vi "Teleop.vi"(10 "Match Info":T1={"Autonomous Elapsed Seconds"=0.0, "TeleOp Elapsed Seconds"=0.0, "Disabled Elapsed Seconds"=0.0, "Visited Autonomous"=FALSE, "Visited TeleOp"=FALSE, "Visited Disabled"=FALSE, "Autonomous Settings"={"Autonomous Style"=enum."Independent", "VI Refnum"=refnum}}, 11 "Call Context":T2) -> ()   [LabVIEW 2016]
doc: "This VI is called for each TeleOp packet received from the DS where the robot is not disabled. It is often used to read from the joysticks and update I/O or to update setpoints for timed control loops. It should complete and return within 20 milliseconds or it may miss DS packets."
uses:
  <vilib>/Rock Robotics/WPI/DriverStation/WPI_DriverStationDerivedRobotMode.ctl
  <vilib>/Rock Robotics/WPI/DriverStation/WPI_DriverStationMatch Info.ctl
  <vilib>/Rock Robotics/WPI/Solenoid/WPI_SolenoidValue.ctl
  <vilib>/Rock Robotics/WPI/Utilities/WPI_GetSetVariantRefNum.vi
  <vilib>/Rock Robotics/WPI/Solenoid/WPI_SolenoidSetEnum.vi
panel:
  out "Gyro Angle":dbl format="%#_13g"
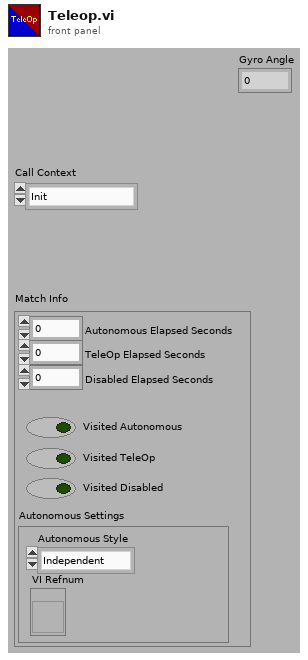
[diagram p1: front panel]
types:
  T1 = typedef "WPI_DriverStationMatch Info.ctl" = cluster{"Autonomous Elapsed Seconds":dbl, "TeleOp Elapsed Seconds":dbl, "Disabled Elapsed Seconds":dbl, "Visited Autonomous":bool, "Visited TeleOp":bool, "Visited Disabled":bool, "Autonomous Settings":cluster{"Autonomous Style":enum16{"Iterative", "Independent"}, "VI Refnum":refnum<vi>}}
  T2 = typedef "WPI_DriverStationDerivedRobotMode.ctl" = enum16{"Init", "Execute", "Stop"}
  T3 = typedef "WPI_SolenoidValue.ctl" = enum16{"Off", "On", "Forward", "Reverse"}
  T4 = typedef "WPI_AccelerometerDevRef.ctl" = cluster{"DevStatus":errorcluster, "Scaling":T5, "Analog Channels":T6, "I2C Bus":T8, "SPI Bus":T9, "Accel Range":T10, "ADXL Axes":T11, "Handle":i32, "Device Address":u8, "Accel Type":enum16{"Analog", "ADXL345 I2C", "ADXL345 SPI", "Internal", "ADXL362 SPI"}}
  T5 = typedef "WPI_AccelerometerScaling.ctl" = cluster{"Gain (VoltsPerG)":dbl, "Center Voltage":dbl}
  T6 = typedef "WPI_AccelerometerAnalogChannels.ctl" = cluster{"X-Axis":T7, "Y-Axis":T7, "Z-Axis":T7}
  T7 = typedef "FPGA_AIChannel.ctl" = enum8{"AI 0", "AI 1", "AI 2", "AI 3", "AI MXP 0", "AI MXP 1", "AI MXP 2", "AI MXP 3", "Invalid"}
  T8 = typedef "i2c_bus.ctl" = enum16{"I2C On-Board", "I2C MXP", "Invalid"}
  T9 = typedef "spi_bus.ctl" = enum16{"SPI On-Board, CS0", "SPI On-Board, CS1", "SPI On-Board, CS2", "SPI On-Board, CS3", "SPI MXP", "Invalid"}
  T10 = typedef "ADXL345 Range.ctl" = u8
  T11 = typedef "WPI_AccelerometerADXL345 Axes.ctl" = cluster{"X-Axis":bool, "Y-Axis":bool, "Z-Axis":bool}
  T12 = cluster{"X-Axis":dbl, "Y-Axis":dbl, "Z-Axis":dbl}
  T13 = typedef "WPI_JoystickDevRef.ctl" = cluster{"Device":T14}
  T14 = typedef "WPI_JoystickDeviceEnum.ctl" = enum16{"USB 0", "USB 1", "USB 2", "USB 3", "USB 4", "USB 5"}
  T15 = typedef "WPI_GyroDevRef.ctl" = cluster{"DevStatus":errorcluster, "Analog Channel":T7, "Offset":dbl, "Gain (VoltsPerDegree/Second)":dbl, "Gyro Type":enum16{"Analog", "XRS450"}, "Handle":i32, "SPI Bus":T9, "Device Found":bool, "Sample Rate":dbl, "Calibrate On Open":bool}
  T16 = typedef "WPI_MotorControlDeviceRef.ctl" = cluster{"DeviceStatus":errorcluster, "Type":T17, "PWM":cluster{"PWM Channel":T18, "DeadBand":T19}, "CAN":cluster{"Device Number":u8, "SetOutput VI Ref":variant, "GetOutput VI Ref":variant, "Enable VI Ref":variant, "Disable VI Ref":variant, "Data":variant}, "Invert":bool}
  T17 = typedef "WPI_MotorControlType.ctl" = enum16{"PWM", "CAN"}
  T18 = typedef "FPGA_DIOPWMChannel.ctl" = enum8{"PWM 0", "PWM 1", "PWM 2", "PWM 3", "PWM 4", "PWM 5", "PWM 6", "PWM 7", "PWM 8", "PWM 9", "PWM MXP 0", "PWM MXP 1", "PWM MXP 2", "PWM MXP 3", "PWM MXP 4", "PWM MXP 5", "PWM MXP 6", "PWM MXP 7", "PWM MXP 8", "PWM MXP 9", "Invalid"}
  T19 = typedef "WPI_PWMDeadband.ctl" = cluster{"Name":string, "maxPositivePwm":i32, "minPositivePwm":i32, "centerPwm":i32, "maxNegativePwm":i32, "minNegativePwm":i32, "angularRange":u16}
  T20 = typedef "WPI_SolenoidDevRef.ctl" = cluster{"DevStatus":errorcluster, "Pneumatics Control Module":u8, "Forward Solenoid Channel":T21, "Reverse Solenoid Channel":T21}
  T21 = typedef "WPI_SolenoidChannel.ctl" = enum8{"Solenoid 0", "Solenoid 1", "Solenoid 2", "Solenoid 3", "Solenoid 4", "Solenoid 5", "Solenoid 6", "Solenoid 7", "Invalid"}
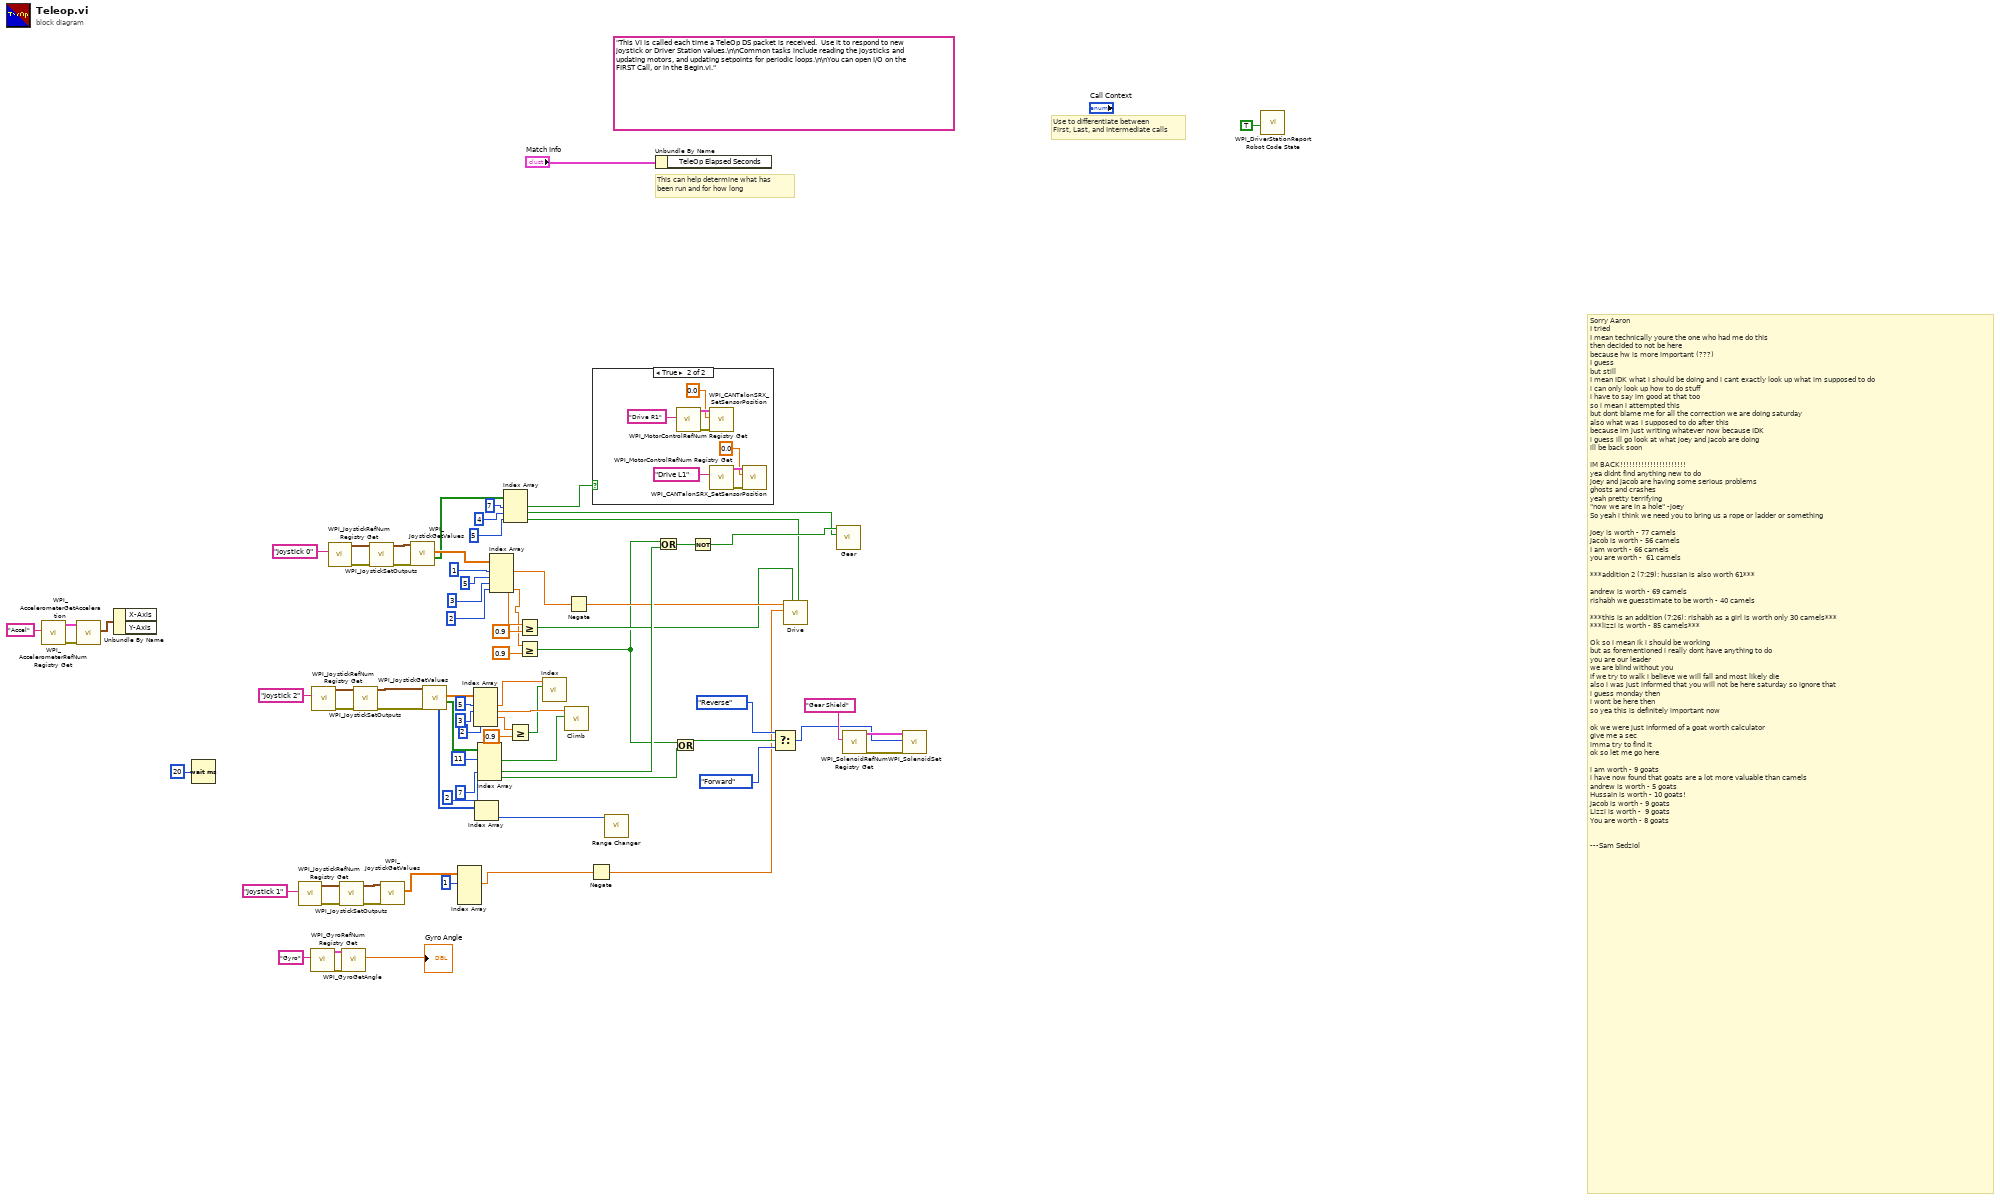
[diagram p0: block diagram]
diagram:
  (unwired) "This VI is called each time a TeleOp DS packet is received.  Use it to respond to new joystick or Driver Station values.\n\nCommon tasks include reading the joysticks and updating motors, and updating setpoints for periodic loops.\n\nYou can open I/O on the FIRST Call, or in the Begin.vi."
  # "Sorry Aaron\nI tried\nI mean technically youre the one who had me do this\nthen decided to not be here\nbecause hw is more important (???)\nI guess\nbut still\nI mean IDK what i should be doing and i cant exactly look up what im supposed to do\ni can only look up how to do stuff\ni have to say im good at that too\nso i mean i attempted this\nbut dont blame me for all the correction we are doing saturday\nalso what was i supposed to do after this\nbecause im just writing whatever now because IDK\ni guess ill go look at what joey and jacob are doing\nill be back soon\n\nIM BACK!!!!!!!!!!!!!!!!!!!!!!\nyea didnt find anything new to do\njoey and jacob are having some serious problems\nghosts and crashes\nyeah pretty terrifying\n\"now we are in a hole\" -joey\nSo yeah i think we need you to bring us a rope or ladder or something\n\nJoey is worth - 77 camels\nJacob is worth - 56 camels\nI am worth - 66 camels\nyou are worth -  61 camels \n\n***addition 2 (7:29): hussian is also worth 61***\n\nandrew is worth - 69 camels\nrishabh we guesstimate to be worth - 40 camels\n\n***this is an addition (7:26): rishabh as a girl is worth only 30 camels***\n***lizzi is worth - 85 camels***\n\nOk so i mean ik i should be working\nbut as forementioned i really dont have anything to do\nyou are our leader\nwe are blind without you\nif we try to walk i believe we will fall and most likely die\nalso i was just informed that you will not be here saturday so ignore that\ni guess monday then\ni wont be here then\nso yea this is definitely important now\n\nok we were just informed of a goat worth calculator\ngive me a sec \nimma try to find it\nok so let me go here\n\ni am worth - 9 goats\ni have now found that goats are a lot more valuable than camels\nandrew is worth - 5 goats\nHussain is worth - 10 goats! \nJacob is worth - 9 goats\nLizzi is worth -  9 goats\nYou are worth - 8 goats\n\n\n---Sam Sedziol"
  # "Use to differentiate between\nFirst, Last, and Intermediate calls"
  # "This can help determine what has\nbeen run and for how long"
  n1 = call <vilib>:"WPI_AccelerometerRefNum Registry Get.vi"("refnum name"="Accel") -> ("error out"=w21:errorcluster, "AccelerometerDevRef"=w20:T4)  [unwired: 9 in]
  n2 = call <vilib>:"WPI_AccelerometerGetAcceleration.vi"("error in"=w21, "AccelerometerDevRef"=w20) -> ("Accelerations"=w22:T12)  [unwired: 7 in, 2 out]
  n3 = Unbundle By Name(w22) -> ()  [unwired: 2 out]
  n4 = Wait (ms)(milliseconds to wait=u32 20) -> ()  [unwired: 1 out]
  n5 = call <vilib>:"WPI_JoystickRefNum Registry Get.vi"("refnum name"="Joystick 1") -> ("error out"=w7:errorcluster, "JoystickDevRef"=w9:T13)  [unwired: 1 in, 8 out]
  n6 = call <vilib>:"WPI_GyroRefNum Registry Get.vi"("refnum name"="Gyro") -> ("error out"=w61:errorcluster, "GyroDevRef"=w60:T15)  [unwired: 9 in]
  n7 = call <vilib>:"WPI_JoystickRefNum Registry Get.vi"("refnum name"="Joystick 2") -> ("error out"=w15:errorcluster, "JoystickDevRef"=w18:T13)  [unwired: 1 in, 8 out]
  n8 = call <vilib>:"WPI_JoystickRefNum Registry Get.vi"("refnum name"="Joystick 0") -> ("error out"=w12:errorcluster, "JoystickDevRef"=w14:T13)  [unwired: 1 in, 8 out]
  n9 = call <vilib>:"WPI_JoystickSetOutputs.vi"("error in (no error)"=w7, "JoystickDevRef"=w9) -> ("error out"=w6:errorcluster, "JoystickDevRef"=w8:T13)  [unwired: 8 in]
  n10 = call <vilib>:"WPI_GyroGetAngle.vi"("error in (no error)"=w61, "GyroDevRef"=w60) -> ("Angle"=→"Gyro Angle":dbl)  [unwired: 6 in, 3 out]
  n11 = call <vilib>:"WPI_JoystickSetOutputs.vi"("error in (no error)"=w15, "JoystickDevRef"=w18) -> ("error out"=w16:errorcluster, "JoystickDevRef"=w17:T13)  [unwired: 8 in]
  n12 = call <vilib>:"WPI_JoystickSetOutputs.vi"("error in (no error)"=w12, "JoystickDevRef"=w14) -> ("error out"=w11:errorcluster, "JoystickDevRef"=w13:T13)  [unwired: 8 in]
  n13 = call <vilib>:"WPI_JoystickGetValues.vi"("error in (no error)"=w6, "JoystickDevRef"=w8) -> ("Axes"=w5:dbl[])  [unwired: 5 in, 4 out]
  n14 = call <vilib>:"WPI_JoystickGetValues.vi"("error in (no error)"=w11, "JoystickDevRef"=w13) -> ("Buttons"=w70:bool[], "Axes"=w74:dbl[])  [unwired: 5 in, 3 out]
  n15 = call <vilib>:"WPI_JoystickGetValues.vi"("error in (no error)"=w16, "JoystickDevRef"=w17) -> ("Buttons"=w71:bool[], "Axes"=w72:dbl[], "POVs"=w50:i16[])  [unwired: 5 in, 2 out]
  n16 = Index Array(array=w5, index #1=1 ("index")) -> (element #1=w3:dbl)  [unwired: 3 in, 3 out]
  n17 = Index Array(array=w72, index #1=5 ("index"), index #2=3 ("index"), index #3=2 ("index")) -> (element #1=w57:dbl, element #2=w66:dbl, element #3=w25:dbl)  [unwired: 1 in, 1 out]
  n18 = Index Array(array=w50) -> (element=w49:i16)  [unwired: 1 in]
  n19 = Index Array(array=w71, index #1=11 ("index"), index #3=7 ("index"), index #4=2) -> (element #1=w54:bool, element #3=w55:bool, element #4=w37:bool)  [unwired: 1 in, 1 out]
  n20 = Index Array(array=w74, index #1=1 ("index"), index #2=5 ("index"), index #3=3 ("index"), index #4=2 ("index")) -> (element #1=w41:dbl, element #3=w35:dbl, element #4=w30:dbl)  [unwired: 1 out]
  n21 = Index Array(array=w70, index #1=7 ("index"), index #2=4 ("index"), index #3=5 ("index")) -> (element #1=w68:bool, element #2=w1:bool, element #3=w27:bool)
  n22 = Greater Or Equal?(x=w25, y=0.9) -> (x >= y?=w23:bool)
  n23 = Greater Or Equal?(x=w35, y=0.9) -> (x >= y?=w31:bool)
  n24 = Greater Or Equal?(x=w30, y=0.9) -> (x >= y?=w29:bool)
  n25 = call "Index.vi"("Shoot"=w23, "Output 2"=w57) -> ()  [unwired: 10 in]
  n26 = call "Climb.vi"("Backwards?"=w54, "Effort"=w66) -> ()  [unwired: 10 in]
  n27 = Negate(x=w41) -> (-x=w36:dbl)
  n28 = Negate(x=w3) -> (-x=w2:dbl)
  n29 = case shown="True" w68 {
    frame False {
    }
    frame True {
      n30 = call <vilib>:"WPI_MotorControlRefNum Registry Get.vi"("refnum name"="Drive R1") -> ("error out"=w80:errorcluster, "MotorControlDevRef"=w79:T16)  [unwired: 9 in]
      n31 = call <vilib>:"WPI_CANTalonSRX_SetSensorPosition.vi"("error in (no error)"=w80, "New Sensor Position"=0.0, "CAN Talon SRX Ref"=w79) -> ()  [unwired: 7 in, 2 out]
      n32 = call <vilib>:"WPI_MotorControlRefNum Registry Get.vi"("refnum name"="Drive L1") -> ("error out"=w82:errorcluster, "MotorControlDevRef"=w83:T16)  [unwired: 9 in]
      n33 = call <vilib>:"WPI_CANTalonSRX_SetSensorPosition.vi"("error in (no error)"=w82, "New Sensor Position"=0.0, "CAN Talon SRX Ref"=w83) -> ()  [unwired: 7 in, 2 out]
    }
  }
  n34 = call "Range Changer.vi"("POV"=w49) -> ()  [unwired: 10 in, 1 out]
  n35 = Unbundle By Name("Match Info") -> ()  [unwired: 1 out]
  n36 = Or(x=w29, y=w55) -> (x .or. y?=w62:bool)
  n37 = Or(x=w29, y=w37) -> (x .or. y?=w38:bool)
  n38 = Not(x=w62) -> (.not. x?=w52:bool)
  n39 = Select(t=WPI_SolenoidValue."Reverse" ("Value"), s=w38, f=WPI_SolenoidValue."Forward" ("Value")) -> (s? t:f=w42:T3)
  n40 = call "Drive.vi"("SwitchDir"=w27, "Slow?"=w31, "Drive R"=w2, "Drive L"=w36) -> ()  [unwired: 8 in]
  n41 = call "Gear.vi"("Gear0?"=w1, "Gear1?"=w52) -> ()  [unwired: 10 in]
  n42 = call <vilib>:"WPI_SolenoidRefNum Registry Get.vi"("refnum name"="Gear Shield") -> ("error out"=w46:errorcluster, "SolenoidDevRef"=w45:T20)  [unwired: 9 in]
  n43 = call-poly <vilib>:"WPI_SolenoidSet.vi"("error in (no error)"=w46, "Value"=w42, "SolenoidDevRef"=w45) -> ()  [unwired: 7 in, 2 out]
  n44 = call <vilib>:"WPI_DriverStationReport Robot Code State.vi"("TeleOp"=TRUE ("Autonomous")) -> ()  [unwired: 10 in, 1 out]
